vi "Status Page Queue Driver.vi"(0 "States":string[](array[string]), 11 "Error in":errorcluster, 13 "Queue Operation":T1) -> (4 "Dequeue Element":string, 15 "Error out":errorcluster)   [LabVIEW 2020, in "INL DNL Test.lvclass"]
doc: "Queue driver to store and execute set of states."
uses:
  INL DNL Test.lvclass
  Typedef/Queue Operation.ctl
  DNL INL Test.lvlib
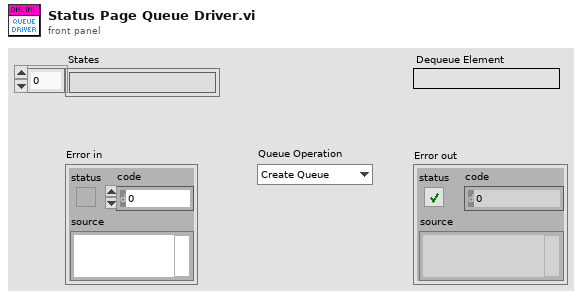
[diagram p1: front panel]
types:
  T1 = typedef "DNL INL Test.lvlib/Queue Operation.ctl" = enum16{"Create Queue", "Enqueue", "Dequeue", "Enstack", "Flush Queue", "Release Queue"}
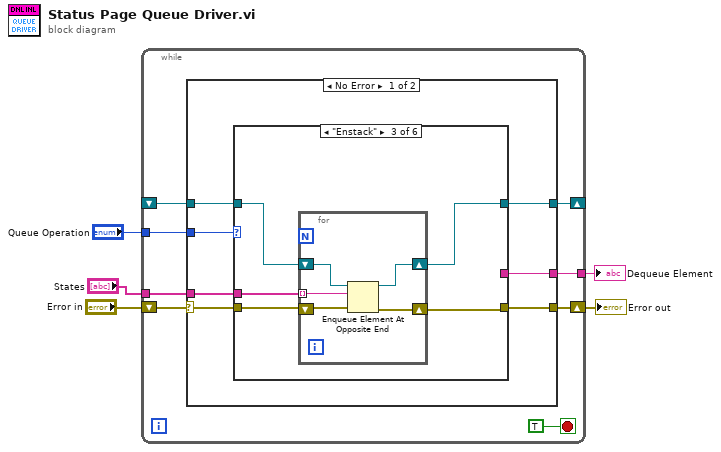
[diagram p0: block diagram]
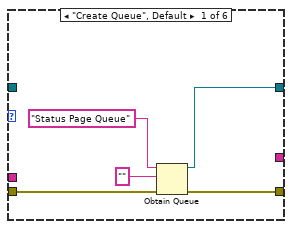
[diagram p2: hidden frame]
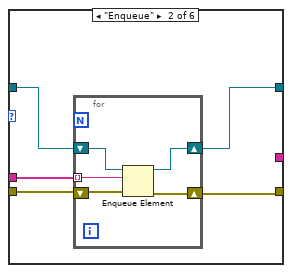
[diagram p3: hidden frame]
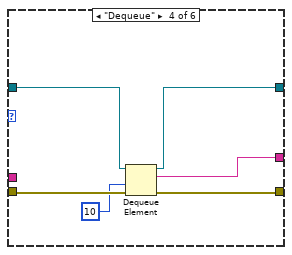
[diagram p4: hidden frame]
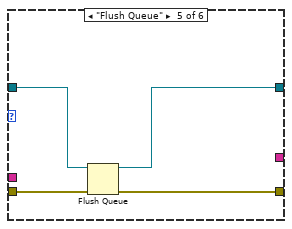
[diagram p5: hidden frame]
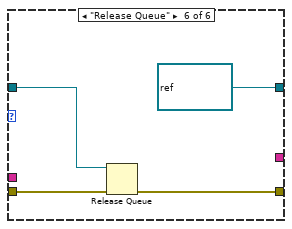
[diagram p6: hidden frame]
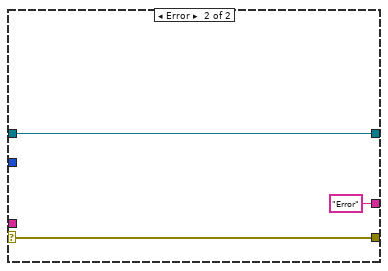
[diagram p7: hidden frame]
diagram:
  n1 = while {
    tunnel: "Queue Operation" -> [w12]
    shift-right: [w9] -> w1
    shift-left: "Error in" -> [w11]
    shift-right: [w10] -> _
    shift-left: _ -> [w8]
    tunnel: "States" -> [w7]
    tunnel: [w6] -> w2
    stop <- TRUE stop-if-true
    n2 = case shown="No Error" w11 {
      selector: w11 -> [w19 w60]
      tunnel: w12 -> [w20 _]
      tunnel: [w18 w61] -> w10
      tunnel: [w17 w60] -> w9
      tunnel: w8 -> [w16 w61]
      tunnel: w7 -> [w15 _]
      tunnel: [w14 "Error"] -> w6
      frame No Error {
        n3 = case shown="\"Enstack\"" w20 {
          tunnel: w19 -> [w25 w30 w40 w51 w55 w59]
          tunnel: [w22 w27 w37 w47 w53 refnum<queue> refnum ("queue out")] -> w18
          tunnel: [w21 w28 w38 w48 w54 w57] -> w17
          tunnel: w16 -> [_ w29 w39 w50 w52 w58]
          tunnel: w15 -> [_ w26 w36 _ _ _]
          tunnel: [_ _ _ w46 _ _] -> w14
          frame "Create Queue", Default {
            n4 = Obtain Queue(name (unnamed)="Status Page Queue", element data type="", error in (no error)=w25) -> (queue out=w22:refnum<queue>, error out=w21:errorcluster)  [unwired: 2 in, 1 out]
          }
          frame "Enqueue" {
            n5 = for {
              shift-right: [w32] -> w28
              shift-left: w30 -> [w35]
              shift-right: [w33] -> w27
              shift-left: w29 -> [w34]
              tunnel: w26 -> [w31] mode=indexing
              n6 = Enqueue Element(queue=w34, element=w31, error in (no error)=w35) -> (queue out=w33:refnum<queue>, error out=w32:errorcluster)  [unwired: 1 in, 1 out]
            }
          }
          frame "Enstack" {
            n7 = for {
              shift-right: [w42] -> w38
              shift-left: w40 -> [w45]
              shift-right: [w43] -> w37
              shift-left: w39 -> [w44]
              tunnel: w36 -> [w41] mode=indexing
              n8 = Enqueue Element At Opposite End(queue=w44, element=w41, error in (no error)=w45) -> (queue out=w43:refnum<queue>, error out=w42:errorcluster)  [unwired: 1 in, 1 out]
            }
          }
          frame "Dequeue" {
            n9 = Dequeue Element(queue=w50, timeout in ms (-1)=10, error in (no error)=w51) -> (queue out=w47:refnum<queue>, element=w46:string, error out=w48:errorcluster)  [unwired: 1 out]
          }
          frame "Flush Queue" {
            n10 = Flush Queue(queue=w52, error in (no error)=w55) -> (queue out=w53:refnum<queue>, error out=w54:errorcluster)  [unwired: 1 out]
          }
          frame "Release Queue" {
            n11 = Release Queue(queue=w58, error in (no error)=w59) -> (error out=w57:errorcluster)  [unwired: 1 in, 2 out]
          }
        }
      }
      frame Error {
      }
    }
  }
  "Dequeue Element" <- w2
  "Error out" <- w1
